vi "move_back.vi"(1 "output cluster":T1) -> (0 "action":T2)   [LabVIEW 2015]
uses:
  ant_base/action_cluster.ctl
  ant_base/actionType_enum.ctl
  Memory.ctl
  ant_base/ant_base.lvclass
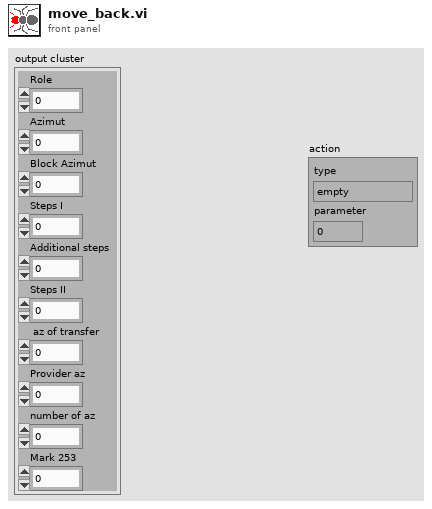
[diagram p1: front panel]
types:
  T1 = typedef "Memory.ctl" = cluster{"Role":i32, "Azimut":i32, "Block Azimut":i32, "Steps I":u32, "Additional steps":i32, "Steps II":u32, " az of transfer":u32, "Provider az":u32, "number of az":u32, "Mark 253":u32}
  T2 = typedef "ant_base.lvclass/action_cluster.ctl" = cluster{"type":T3, "parameter":dbl}
  T3 = typedef "ant_base.lvclass/actionType_enum.ctl" = enum8{"empty", "move", "take", "put", "mark"}
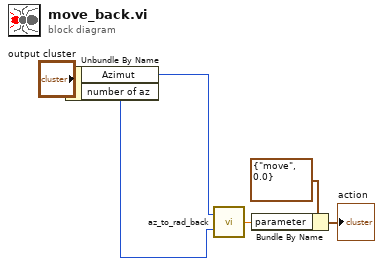
[diagram p0: block diagram]
diagram:
  n1 = Unbundle By Name("output cluster") -> ("Azimut"=w2:i32, "number of az"=w1:u32)
  n2 = call "az_to_rad_back.vi"("az quantity"=w1, "az"=w2) -> ("rad"=w4:dbl)
  n3 = Bundle By Name(cluster=T2 {"type"=enum."move", "parameter"=0.0} ("action"), "parameter"=w4) -> (→"action":T2)
